vi "New Results (to override).vi"(7 "Image Nr.":i32, 8 "error in (no error)":errorcluster, 9 "Results In":refnum<class "Analyze Results Base.lvclass">[](array[class]), 10 "Parameters":refnum<class "Analyze Parameter Base.lvclass">[](array[class]), 11 "HIJ Single Cam App Demo In":refnum<class "HIJ Vision App Fluence and Energy Camera.lvclass">) -> (0 "error out":errorcluster, 3 "HIJ Single Cam App Demo Out":refnum<class "HIJ Vision App Fluence and Energy Camera.lvclass">)   [LabVIEW 2014, in "HIJ Vision App Fluence and Energy Camera.lvlib" / "HIJ Vision App Fluence and Energy Camera.lvclass"]
uses:
  HIJ Vision App Fluence and Energy Camera.lvclass
  Analyze/Results and Overlays/Results Base/Analyze Results Base.lvclass
  Analyze/Analyze Parameter/Analyze Parameter Base/Analyze Parameter Base.lvclass
  <vilib>/ActorFramework/Actor/Actor.lvclass/Actor.ctl
  HIJ Vision App Fluence and Energy Camera.lvclass/HIJ Vision App Fluence and Energy Camera.ctl
  Abstract Messages/Publish Analyze Results Msg/Publish Analyze Results Msg.lvclass/Publish Analyze Results Msg.ctl
  <vilib>/ActorFramework/Message Enqueuer/Message Enqueuer.lvclass/Message Enqueuer.ctl
  Analyze/Results and Overlays/Results Fluence and Energy/Analyze Results Fluence and Energy.lvclass
  Analyze/Results and Overlays/Results Total Counts/Analyze Results Total Counts.lvclass/Analyze Results Total Counts.ctl
  Analyze/Results and Overlays/Results Total Counts/Read Total Counts.vi
  <vilib>/ActorFramework/Message Enqueuer/Enqueue.vi
  <vilib>/ActorFramework/Message Priority Queue/Priority Enqueue.vi
  HIJ Vision Camera App/HIJ Vision Camera App/HIJ Vision Camera App.lvclass
  <vilib>/ActorFramework/Message Enqueuer/Message Enqueuer.lvclass
  <vilib>/ActorFramework/Actor/Actor.lvclass
  Abstract Messages/Publish Analyze Results Msg/Publish Analyze Results Msg.lvclass
  Analyze/Results and Overlays/Results Energy/Analyze Results Energy.lvclass
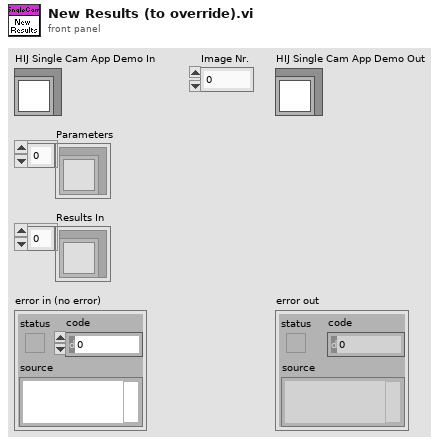
[diagram p1: front panel]
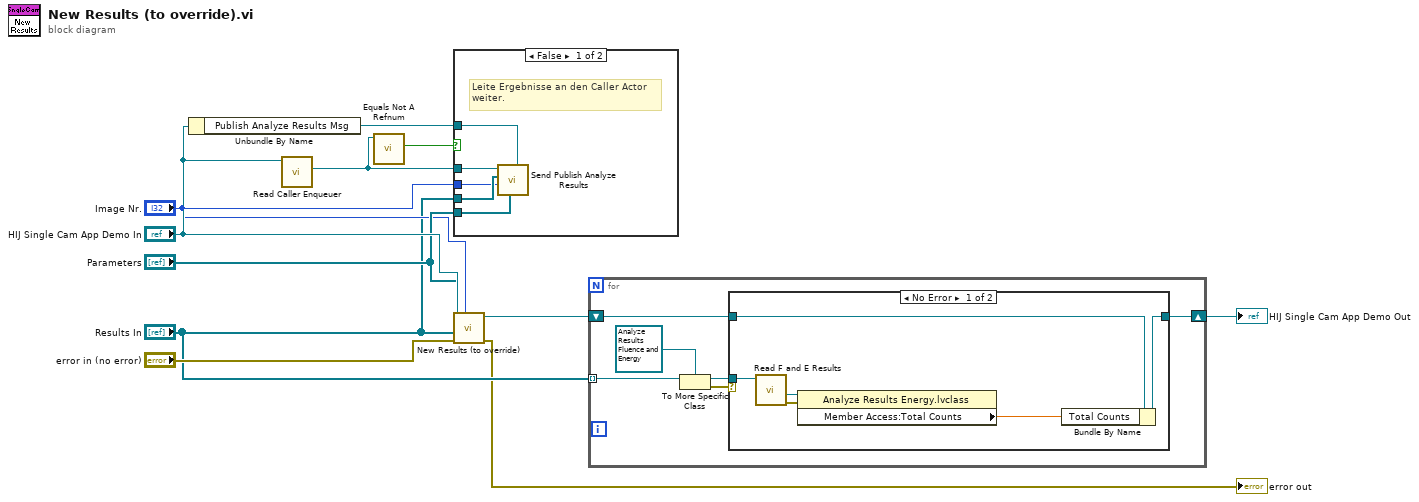
[diagram p0: block diagram]
diagram:
  n1 = Unbundle By Name("HIJ Single Cam App Demo In") -> ("Publish Analyze Results Msg"=w9:refnum<class "Publish Analyze Results Msg.lvclass">)
  n2 = call <vilib>:"Read Caller Enqueuer.vi"("Actor"="HIJ Single Cam App Demo In") -> ("Caller Enqueuer"=w7:refnum<class "Message Enqueuer.lvclass">)  [unwired: 10 in]
  n3 = call <vilib>:"Equals Not A Refnum.vi"("Message Enqueuer"=w7) -> ("Not a refnum?"=w6:bool)  [unwired: 10 in]
  n4 = case shown="False" w6 {
    tunnel: w9 -> [w16 _]
    tunnel: "Results In" -> [w15 _]
    tunnel: "Parameters" -> [w14 _]
    tunnel: w7 -> [w13 _]
    tunnel: "Image Nr." -> [w12 _]
    frame False {
      # "Leite Ergebnisse an den Caller Actor\nweiter."
      n5 = call "Send Publish Analyze Results.vi"("Message Type"=w16, "Parameters"=w14, "Image Nr."=w12, "Results In"=w15, "Message Enqueuer"=w13) -> ()  [unwired: 5 in, 2 out]
    }
    frame True {
    }
  }
  n6 = call-parent "New Results (to override).vi"("Image Nr."="Image Nr.", "error in (no error)"="error in (no error)", "Results In"="Results In", "Parameters"="Parameters", "HIJ Vision Camera App In"="HIJ Single Cam App Demo In") -> ("error out"=→"error out":errorcluster, "HIJ Vision Camera App Out"=w2:refnum<class "HIJ Vision App Fluence and Energy Camera.lvclass">)  [unwired: 5 in]
  n7 = for {
    tunnel: "Results In" -> [w22] mode=indexing
    shift-right: [w19] -> w3
    shift-left: w2 -> [w20]
    n8 = To More Specific Class(target class=refnum<class "Analyze Results Fluence and Energy.lvclass"> refnum ("Analyze Results Fluence and Energy.lvclass"), reference=w22) -> (specific class reference=w18:refnum<class "Analyze Results Fluence and Energy.lvclass">, error out=w17:errorcluster)  [unwired: 1 in]
    n9 = case shown="No Error" w17 {
      tunnel: w20 -> [w28 w29]
      tunnel: [w27 w29] -> w19
      tunnel: w18 -> [w26 _]
      frame No Error {
        n10 = call "Read F and E Results.vi"("Analyze Results Fluence and Energy in"=w26) -> ("error out"=w23:errorcluster, "Energy"=w25:refnum<class "Analyze Results Energy.lvclass">)  [unwired: 7 in, 2 out]
        n11 = property class="Analyze Results Energy.lvclass"(reference=w25, error in=w23) -> ("Member Access:Total Counts"=w24:dbl)  [unwired: 2 out]
        n12 = Bundle By Name(cluster=w28, "Total Counts"=w24) -> (w27:refnum<class "HIJ Vision App Fluence and Energy Camera.lvclass">)
      }
      frame Error {
      }
    }
  }
  "HIJ Single Cam App Demo Out" <- w3
